vi "PopConnection.vi"(0 "reference":refnum<class "VdTcpIP.lvclass">, 1 "ms timeout (-1=forever)":i32=-1, 5 "error in (no error)":errorcluster) -> (14 "reference out":refnum<class "VdTcpIP.lvclass">, 15 "NewSocketConnection":refnum<class "VdTcpIP.lvclass">, 19 "error out":errorcluster)   [LabVIEW 2020, in "VdTcpIP.lvclass"]
doc: "Pops a connection from the connection array\nIf no cennection found it will wait untile timeout."
uses:
  VdTcpIP.lvclass
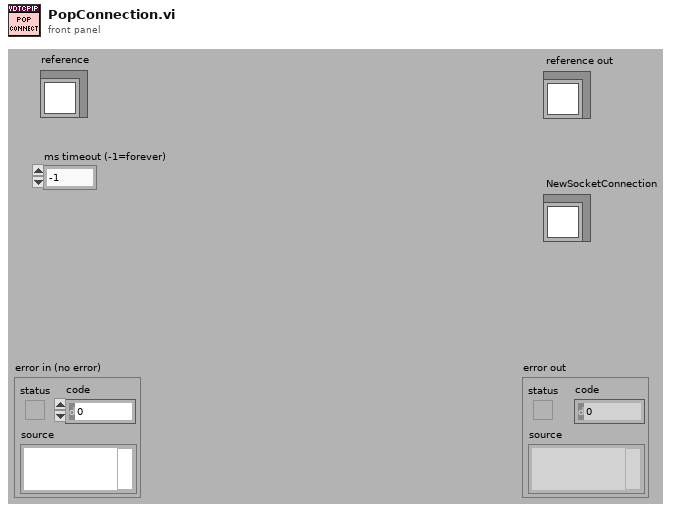
[diagram p1: front panel]
types:
  T1 = typedef "VdTcpIP.lvclass/ObjectAttributes.ctl" = cluster{"IP-Address":string, "Port":u16, "Connection":refnum<k5>, "Listener":refnum<k5>, "ListenerConnection":refnum<k5>, "Listner":bool, "ListnerProcessRunning":bool, "InConnections":refnum<k5>[], "InConnectionsIP":string[], "InConnectionAdded":refnum<notifier>, "RunVIOnNewConnection":variant, "DataToNewConnectionVI":cluster{"ControlName":string, "ControlValue":variant}[], "WebServicesURL_Location(http://...)":string, "WebServicesPostWebPage(*.asmx)":string, "Semaphore":T2, "AutoReConnectTimes":i32, "AutoReConnectInterval(ms)":i32, "ConnectionTimeout":i32}
  T2 = typedef "Semaphore RefNum" = refnum<k1>
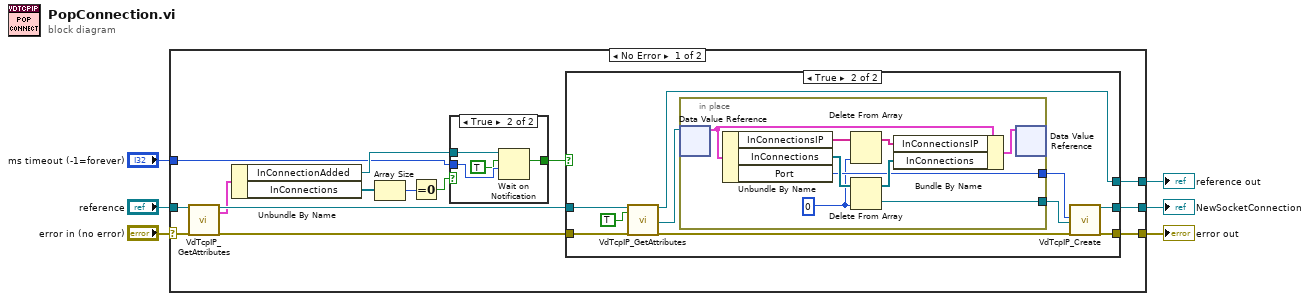
[diagram p0: block diagram]
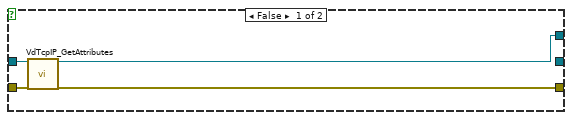
[diagram p2: hidden frame]
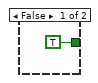
[diagram p3: hidden frame]
diagram:
  n1 = case shown="No Error" "error in (no error)" {
    selector: "error in (no error)" -> [w9 w49]
    tunnel: "reference" -> [w20 w50]
    tunnel: [w11 w49] -> w4
    tunnel: [w19 w50] -> w3
    tunnel: "ms timeout (-1=forever)" -> [w13 _]
    tunnel: [w12 _] -> w1
    frame No Error {
      n2 = call "VdTcpIP_GetAttributes.vi"("reference in"=w20, "error in (no error)"=w9) -> ("reference out"=w18:refnum<class "VdTcpIP.lvclass">, "Data"=w7:T1, "error out"=w10:errorcluster)  [unwired: 1 in, 14 out]
      n3 = Unbundle By Name(w7) -> ("InConnectionAdded"=w14:refnum<notifier>, "InConnections"=w17:refnum<k5>[])
      n4 = Array Size(array=w17) -> (size(s)=w16:i32)
      n5 = Equal To 0?(x=w16) -> (x = 0?=w15:bool)
      n6 = case shown="True" w15 {
        tunnel: w14 -> [_ w48]
        tunnel: w13 -> [_ w47]
        tunnel: [TRUE w45] -> w8
        frame False {
        }
        frame True {
          n7 = Wait on Notification(notifier=w48, ignore previous (F)=TRUE, timeout in ms (-1)=w47) -> (notification=w45:bool)  [unwired: 1 in, 3 out]
        }
      }
      n8 = case shown="True" w8 {
        tunnel: [w23 w34] -> w19
        tunnel: w18 -> [w24 w33]
        tunnel: [_ w32] -> w12
        tunnel: [w22 w30] -> w11
        tunnel: w10 -> [w21 w29]
        frame False {
          n9 = call "VdTcpIP_GetAttributes.vi"("reference in"=w24, "error in (no error)"=w21) -> ("reference out"=w23:refnum<class "VdTcpIP.lvclass">, "error out"=w22:errorcluster)  [unwired: 1 in, 15 out]
        }
        frame True {
          n10 = call "VdTcpIP_GetAttributes.vi"("reference in"=w33, "OnlyGetDvrReference(False)"=TRUE, "error in (no error)"=w29) -> ("reference out"=w34:refnum<class "VdTcpIP.lvclass">, "DataRef"=w27:refnum<data-value>, "error out"=w31:errorcluster)  [unwired: 13 in, 1 out]
          n11 = in-place {
            in-place-border: [w37] -> w26
            in-place-border: [w36] -> w25
            w35 = 0 ("index")
            n12 = in-place-dvr #1(w27) -> (w43:T1)  [unwired: 1 out]
            n13 = Unbundle By Name(w43) -> ("InConnectionsIP"=w39:string[], "InConnections"=w38:refnum<k5>[], "Port"=w37:u16)
            n14 = Delete From Array(array=w39, index=w35) -> (array with subset deleted=w42:string[])  [unwired: 1 in, 1 out]
            n15 = Delete From Array(array=w38, index=w35) -> (deleted portion=w36:refnum<k5>, array with subset deleted=w41:refnum<k5>[])  [unwired: 1 in]
            n16 = Bundle By Name(cluster=w43, "InConnectionsIP"=w42, "InConnections"=w41) -> (w40:T1)
            n17 = in-place-dvr #1(w40) -> ()  [unwired: 2 out]
          }
          n18 = call "VdTcpIP_Create.vi"("Port"=w26, "Connection"=w25, "error in (no error)"=w31) -> ("reference out"=w32:refnum<class "VdTcpIP.lvclass">, "error out"=w30:errorcluster)  [unwired: 4 in, 11 out]
        }
      }
    }
    frame Error {
    }
  }
  "reference out" <- w3
  "error out" <- w4
  "NewSocketConnection" <- w1
